vi "HostTestSimpleCounter.vi"() -> ()   [LabVIEW 2014]
uses:
  <vilib>/rvi/interface/nirviOpenFPGA/nirviOpenFPGA.xnode
  <vilib>/rvi/interface/nirviCloseFPGA/nirviCloseFPGA.xnode
  <vilib>/rvi/interface/nirviReadWriteControl/nirviReadWriteControl.xnode
  <vilib>/rvi/interface/nirviMethod/nirviMethod.xnode
  <vilib>/FPGAPlugInAG/Dynamic/niLvFpga_ReadFifo_Dynamic.vi
  <vilib>/rvi/errors/niLvFpgaMergeErrorWithErrorCode.vi
  <vilib>/rvi/interface/Simulation/niFpgaSimulationCallBeginRW.vi
  <vilib>/rvi/errors/niLvFpgaAdjustHostInterfaceError.vi
  <vilib>/FPGAPlugInAG/Dynamic/niLvFpga_Run_Dynamic.vi
  FPGA Bitfiles/TiTaProj_DAF_SPTopLevel_1.lvbitx
  SimpleCounter/SPTopLevel.vi
  <vilib>/FPGAPlugInAG/Dynamic/niLvFpga_ConfigureFifo_Dynamic.vi
  <vilib>/FPGAPlugInAG/Dynamic/niLvFpga_StartFifo_Dynamic.vi
  <vilib>/FPGAPlugInAG/Dynamic/niLvFpga_Close_Dynamic.vi
panel:
  in  "SetVolt":bool
  in  "SetVolt":u32 format="%024b"
  in  "heinzingerControl":T1(ring)
  out "Actual Depth":u32
  in  "Requested Depth":u32
  out "Overflow":bool
  out "reading .. Elements":u32
  out "output array":u32[](array[numeric]) format="%032b"
  out "Elements Remaining":u32
  in  "stop":bool
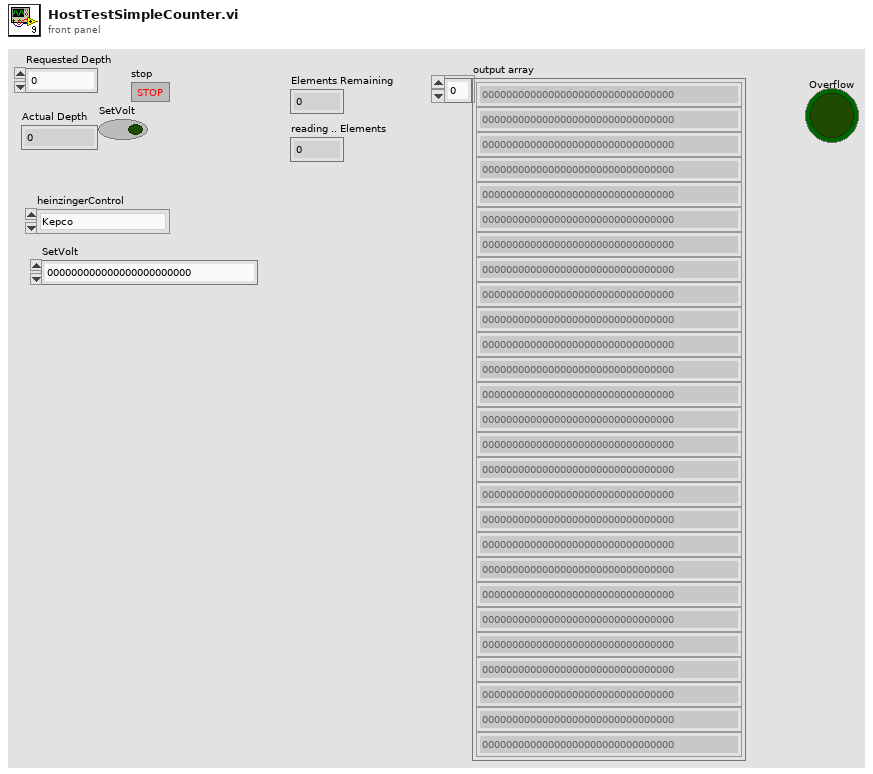
[diagram p1: front panel]
types:
  T1 = enum8{"Kepco", "Heinzinger0", "Heinzinger1", "Heinzinger2"}
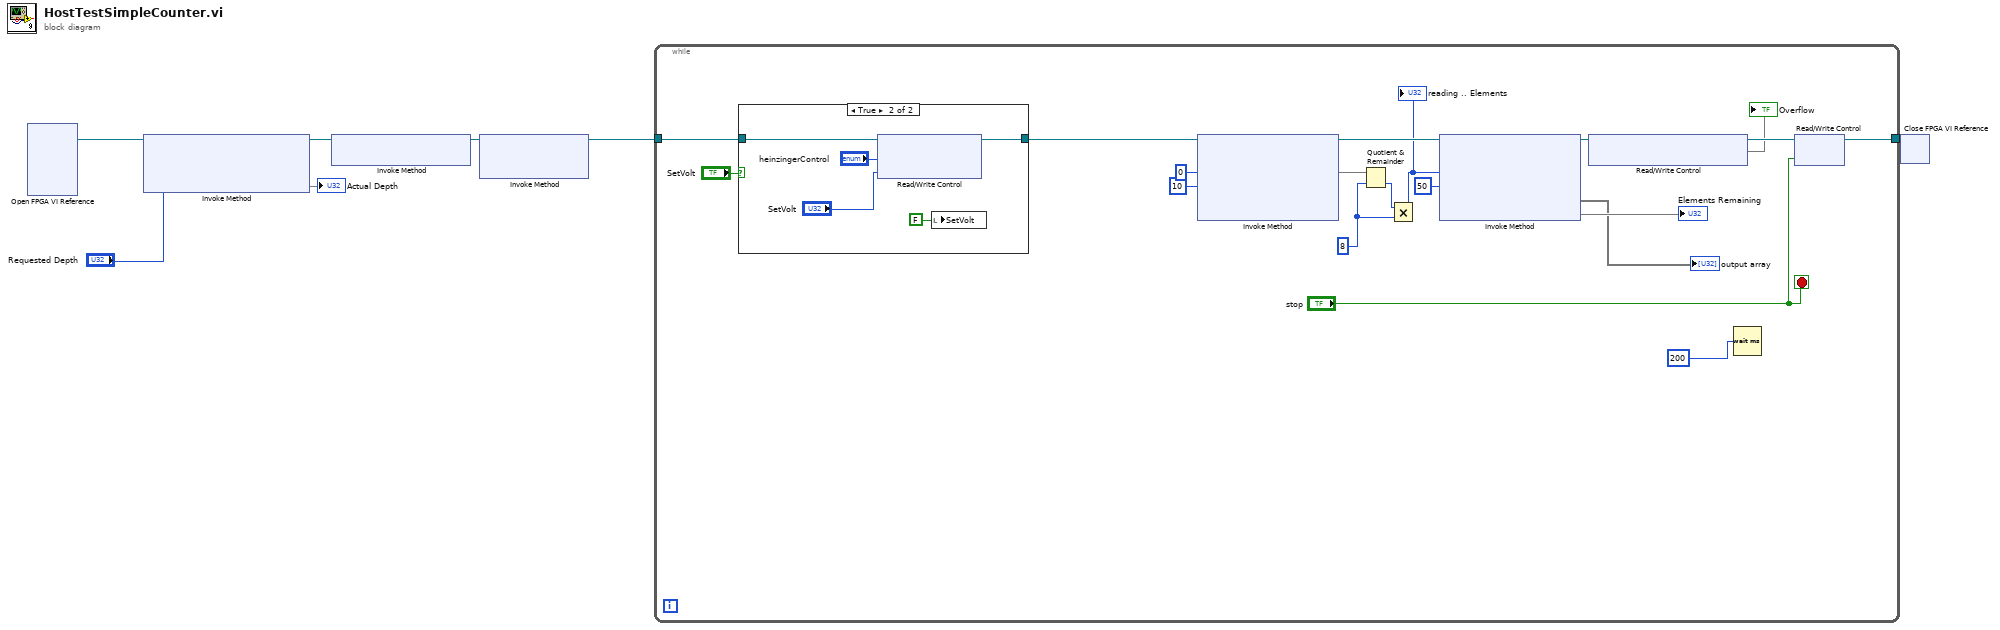
[diagram p0: block diagram]
diagram:
  n1 = xnode "Open FPGA VI Reference"() -> ("FPGA VI Reference Out"=w4:refnum<k20>)  [unwired: 2 in, 1 out]
  n2 = xnode "Invoke Method"("FPGA VI Reference In"=w4, "Requested Depth"="Requested Depth") -> ("FPGA VI Reference Out"=w3:refnum<k20>, "Actual Depth"=→"Actual Depth")  [unwired: 1 in, 1 out]
  n3 = xnode "Invoke Method"("FPGA VI Reference In"=w3) -> ("FPGA VI Reference Out"=w6:refnum<k20>)  [unwired: 1 in, 1 out]
  n4 = xnode "Invoke Method"("FPGA VI Reference In"=w6) -> ("FPGA VI Reference Out"=w5:refnum<k20>)  [unwired: 2 in, 1 out]
  n5 = while {
    tunnel: w5 -> [w22]
    tunnel: [w23] -> w7
    stop <- "stop" stop-if-true
    w15 = u32 8 ("y")
    n6 = case shown="True" "SetVolt" {
      tunnel: w22 -> [w27 w32]
      tunnel: [w27 w31] -> w9
      frame False {
      }
      frame True {
        n7 = xnode "Read/Write Control"("FPGA VI Reference In"=w32, "heinzingerControl"="heinzingerControl", "SetVolt"="SetVolt") -> ("FPGA VI Reference Out"=w31:refnum<k20>)  [unwired: 1 in, 1 out]
        n8 = local write "SetVolt"(FALSE ("SetVolt")) -> ()
      }
    }
    n9 = xnode "Invoke Method"("FPGA VI Reference In"=w9, "Number of Elements"=u32 0, "Timeout (ms)"=10) -> ("FPGA VI Reference Out"=w25:refnum<k20>, "Elements Remaining"=w20)  [unwired: 1 in, 2 out]
    n10 = Quotient & Remainder(x=w20, y=w15) -> (floor(x/y)=w14:u32)  [unwired: 1 out]
    n11 = Multiply(x=w14, y=w15) -> (x*y=w10:u32)
    "reading .. Elements" <- w10
    n12 = xnode "Invoke Method"("FPGA VI Reference In"=w25, "Number of Elements"=w10, "Timeout (ms)"=50) -> ("FPGA VI Reference Out"=w24:refnum<k20>, "Data"=→"output array":void[], "Elements Remaining"=→"Elements Remaining")  [unwired: 1 in, 1 out]
    n13 = xnode "Read/Write Control"("FPGA VI Reference In"=w24) -> ("FPGA VI Reference Out"=w13:refnum<k20>, "simpleCounterWriteOverflow"=→"Overflow")  [unwired: 1 in, 1 out]
    n14 = Wait (ms)(milliseconds to wait=u32 200) -> ()  [unwired: 1 out]
    n15 = xnode "Read/Write Control"("FPGA VI Reference In"=w13, "stop"="stop") -> ("FPGA VI Reference Out"=w23:refnum<k20>)  [unwired: 1 in, 1 out]
  }
  n16 = xnode "Close FPGA VI Reference"("FPGA VI Reference In"=w7) -> ()  [unwired: 1 in, 1 out]
